vi "PicoScope3000aGetTimebase2.vi"(4 "Number of Samples":u32, 6 "Memory Segment":u32, 7 "Acquisition Settings":T1={"preTriggerSamples"=0, "postTriggerSamples"=5000000, "timebase"=5} {"postTriggerSamples" format="%_6p"; "preTriggerSamples" format="%_6p"}, 8 "error in (no error)":errorcluster, 11 "handle in":i16) -> (0 "error out":errorcluster, 3 "handle out":i16, 5 "Properties Panel":T2 {"Max Total Capture Time Available (sec)" format="%.3p"; "Sample Frequency" format="%.3p"; "Sample Rate" format="%.3p"; "Max Samples Available" format="%.3p"; "Total Capture Time (sec)" format="%.3p"})   [LabVIEW 2010]
uses:
  ps3000a.dll
  shared/Acquisition Settings.ctl
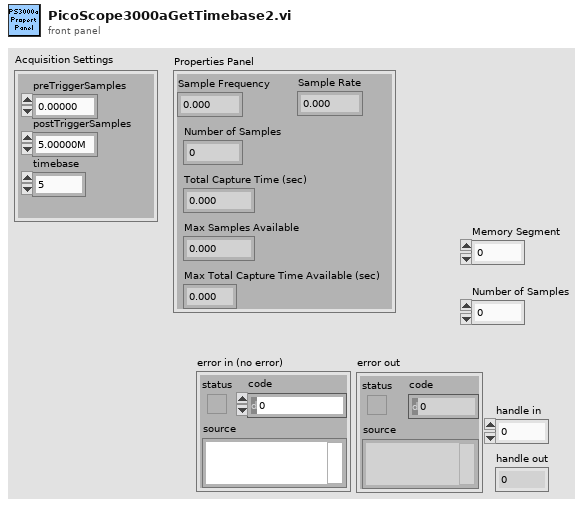
[diagram p1: front panel]
types:
  T1 = typedef "Acquisition Settings.ctl" = cluster{"preTriggerSamples":u64, "postTriggerSamples":u64, "timebase":u32}
  T2 = cluster{"Sample Frequency":sgl, "Sample Rate":sgl, "Max Samples Available":i32, "Number of Samples":u32, "Total Capture Time (sec) ":sgl, "Max Total Capture Time Available (sec)":sgl}
  T3 = cluster{sgl, sgl, "maxSamples":i32, "Number of Samples":u32, sgl, sgl}
  T4 = cluster{"status":bool, "code":u32, "source":string}
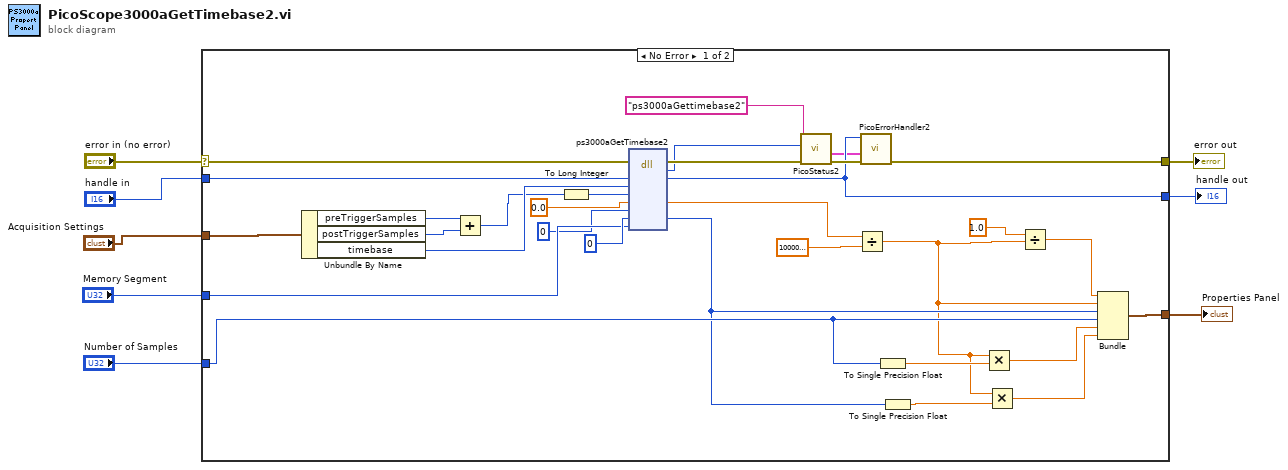
[diagram p0: block diagram]
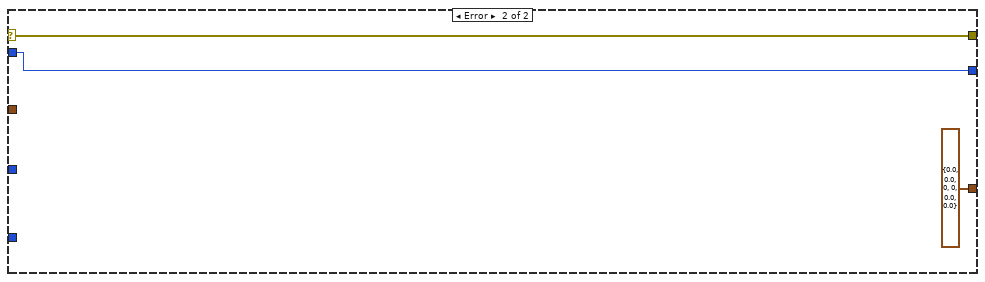
[diagram p2: hidden frame]
diagram:
  n1 = case shown="No Error" "error in (no error)" {
    selector: "error in (no error)" -> [w13 w42]
    tunnel: [w12 w42] -> w8
    tunnel: [w10 w41] -> w7
    tunnel: "Memory Segment" -> [w30 _]
    tunnel: "Number of Samples" -> [w25 _]
    tunnel: "handle in" -> [w29 w41]
    tunnel: "Acquisition Settings" -> [w28 _]
    tunnel: [w21 T3 {0.0, 0.0, "maxSamples"=0, "Number of Samples"=0, 0.0, 0.0}] -> w2
    frame No Error {
      n2 = Unbundle By Name(w28) -> ("preTriggerSamples"=w34:u64, "postTriggerSamples"=w35:u64, "timebase"=w36:u32)
      n3 = Add(x=w34, y=w35) -> (x+y=w15:u64)
      n4 = To Long Integer(number=w15) -> (32bit integer=w16:i32)
      n5 = dll-call lib="ps3000a.dll" fn="ps3000aGetTimebase2"(error in=w13, "handle"=w29, "timebase"=w36, "noSamples"=w16, "timeIntervalNanoseconds"=sgl 0.0, "oversample"=i16 0, "maxSamples"=0, "segmentIndex"=w30) -> (error out=w37:errorcluster, "PICO_STATUS"=w31:u32, "handle"=w10:i16, "timeIntervalNanoseconds"=w38:sgl, "maxSamples"=w23:i32)  [unwired: 6 in, 1 out]
      n6 = call "PicoStatus2.vi"("PICO source"="ps3000aGettimebase2" ("source"), "Error in"=w37, "PICO STATUS"=w31) -> ("error out"=w11:errorcluster, "PICO_STATUS out"=w9:T4)  [unwired: 5 in]
      n7 = Divide(x=w38, y=sgl 1000000000.0) -> (x/y=w20:sgl)
      n8 = call "PicoErrorHandler2.vi"("error in (no error)"=w11, "PICO_STATUS in"=w9, "handle In"=w10) -> ("error out"=w12:errorcluster)  [unwired: 8 in]
      n9 = To Single Precision Float(number=w25) -> (single precision float=w27:sgl)
      n10 = To Single Precision Float(number=w23) -> (single precision float=w24:sgl)
      n11 = Multiply(x=w20, y=w27) -> (x*y=w26:sgl)
      n12 = Multiply(x=w20, y=w24) -> (x*y=w22:sgl)
      n13 = Divide(x=sgl 1.0, y=w20) -> (x/y=w18:sgl)
      n14 = Bundle(w18, w20, "maxSamples"=w23, "Number of Samples"=w25, w26, w22) -> (w21:T3)  [unwired: 1 in]
    }
    frame Error {
    }
  }
  "error out" <- w8
  "handle out" <- w7
  "Properties Panel" <- w2
